vi "ISO8601 DateString to Timestamp.vi"(9 "Strict ISO? (T)":bool=TRUE, 11 "ISO8601 Date String":string) -> (1 "valid?":bool, 2 "ISO Format":T1, 3 "Timestamp":timestamp)   [LabVIEW 2018]
uses:
  ISO8601 Date Formats.ctl
  <vilib>/Utility/miscctls.llb/LVDateTimeRec.ctl
  Timestamp to ISO8601 Day.vi
  isLeapYear (integer).vi
  <vilib>/regexp/Match Regular Expression.xnode
  DateTime.ISO8601.lvclass
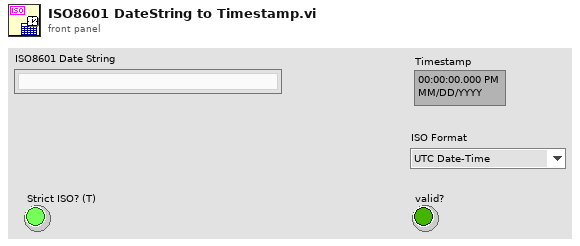
[diagram p1: front panel]
types:
  T1 = typedef "ISO8601 Date Formats.ctl" = enum16{"UTC Date-Time", "Date", "Calendar Month", "Week", "Week-Day", "Month-Day", "Ordinal Date"}
  T2 = typedef "LVDateTimeRec.ctl" = cluster{"fractional second":dbl, "second":i32, "minute":i32, "hour":i32, "day of month":i32, "month":i32, "year":i32, "day of week":i32, "day of year":i32, "DST":i32}
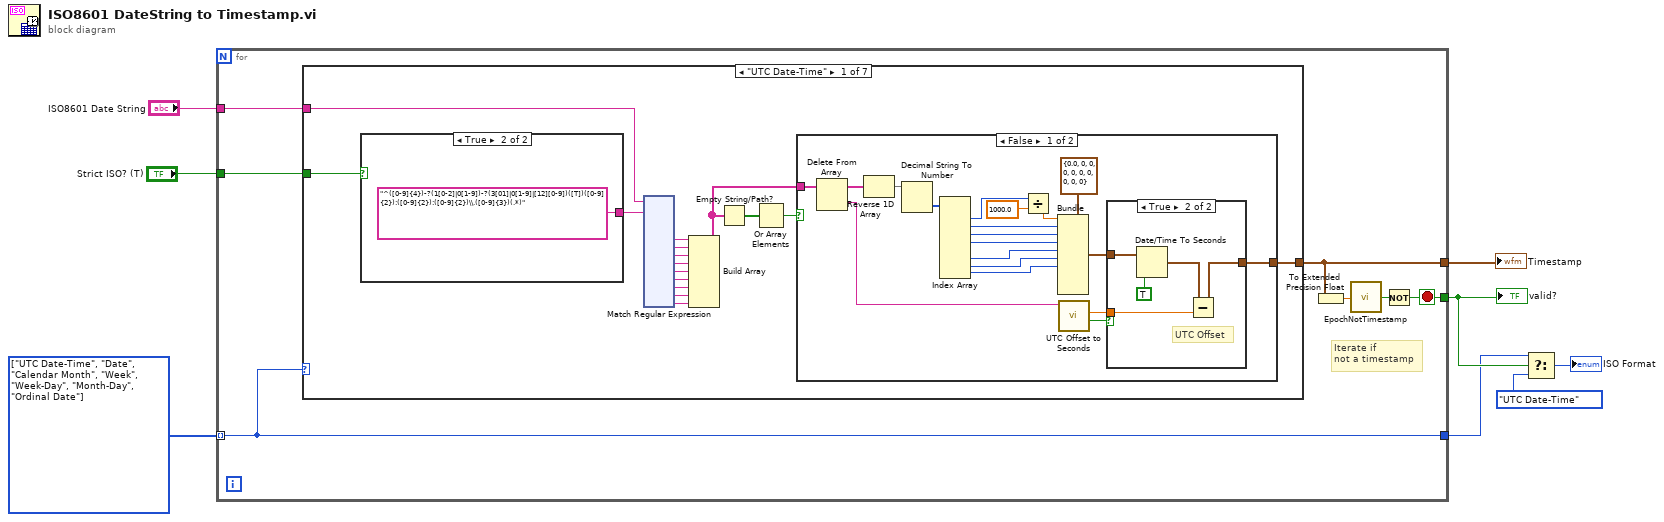
[diagram p0: block diagram]
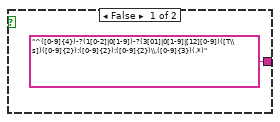
[diagram p4: hidden frame]
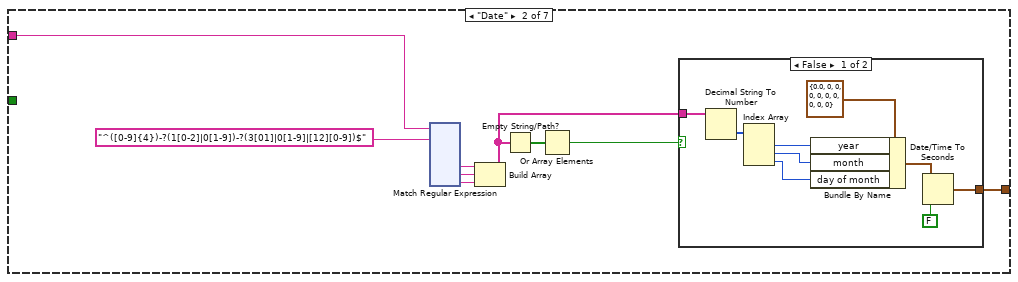
[diagram p5: hidden frame]
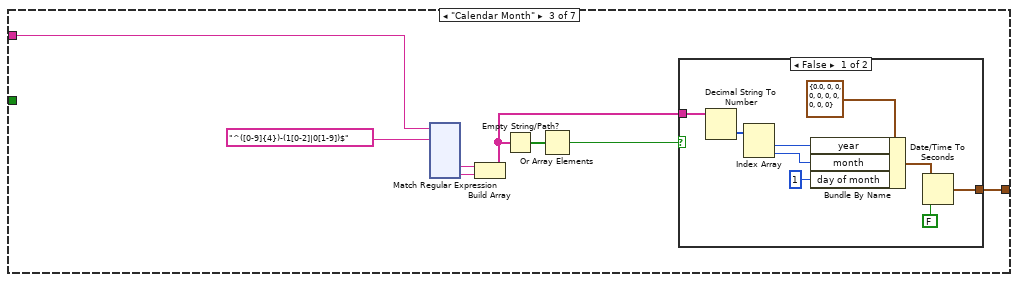
[diagram p7: hidden frame]
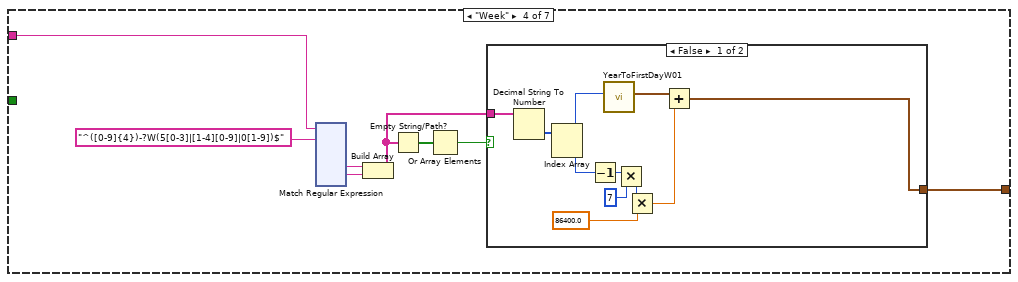
[diagram p9: hidden frame]
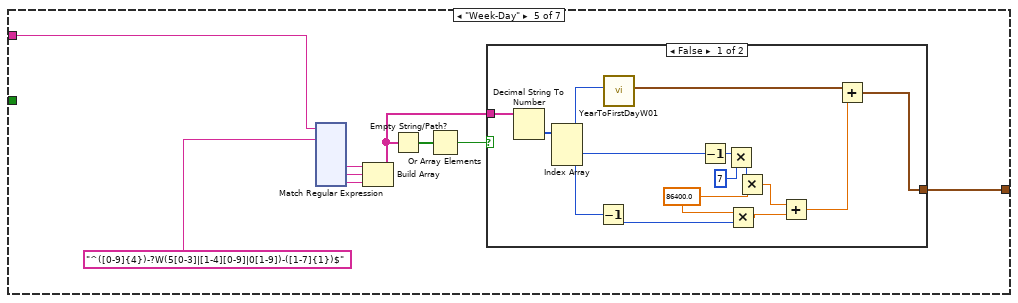
[diagram p11: hidden frame]
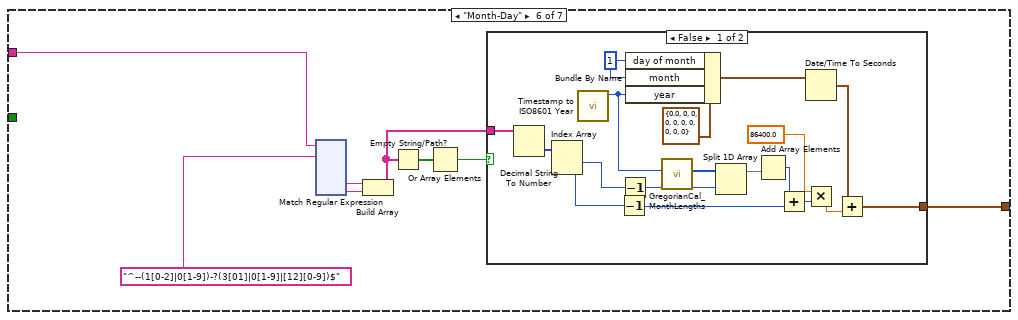
[diagram p13: hidden frame]
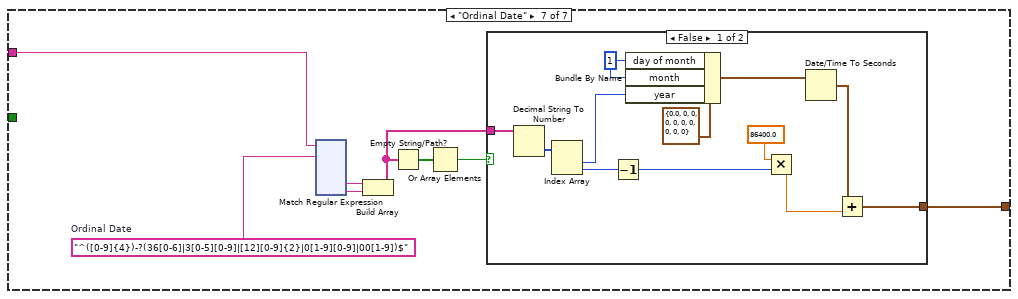
[diagram p15: hidden frame]
diagram:
  w6 = T1[] [enum."UTC Date-Time", enum."Date", enum."Calendar Month", enum."Week", enum."Week-Day", enum."Month-Day", enum."Ordinal Date"] items=["UTC Date-Time", "Date", "Calendar Month", "Week", "Week-Day", "Month-Day", "Ordinal Date"]
  n1 = for {
    tunnel: "ISO8601 Date String" -> [w15]
    tunnel: [w14] -> w7
    tunnel: [w11] -> w5
    tunnel: [w10] -> w4
    tunnel: w6 -> [w10] mode=indexing
    tunnel: "Strict ISO? (T)" -> [w9]
    stop <- w11 stop-if-true
    # "Iterate if\nnot a timestamp"
    n2 = case shown="\"UTC Date-Time\"" w10 {
      tunnel: w15 -> [w18 w184 w320 w454 w592 w733 w876]
      tunnel: w9 -> [w31 _ _ _ _ _ _]
      tunnel: [w30 w190 w325 w459 w597 w738 w881] -> w14
      frame "UTC Date-Time" {
        n3 = case shown="True" w31 {
          tunnel: ["^([0-9]{4})-?(1[0-2]|0[1-9])-?(3[01]|0[1-9]|[12][0-9])([T\\s])([0-9]{2}):([0-9]{2}):([0-9]{2})\\.([0-9]{3})(.*)" ("regular expression") "^([0-9]{4})-?(1[0-2]|0[1-9])-?(3[01]|0[1-9]|[12][0-9])([T])([0-9]{2}):([0-9]{2}):([0-9]{2})\\.([0-9]{3})(.*)" ("regular expression")] -> w17
          frame False {
          }
          frame True {
          }
        }
        n4 = xnode "Match Regular Expression"("input string"=w18, "regular expression"=w17) -> ("submatch 1"=w29:string, "submatch 2"=w28:string, "submatch 3"=w27:string, "submatch 4"=w26:string, "submatch 5"=w25:string, "submatch 6"=w24:string, "submatch 7"=w23:string, "submatch 8"=w22:string, "submatch 9"=w21:string)  [unwired: 4 in, 5 out]
        n5 = Build Array(w29, w28, w27, w26, w25, w24, w23, w22, w21) -> (w16:string[])
        n6 = Empty String/Path?(string/path=w16) -> (empty?=w20:bool[])
        n7 = Or Array Elements(Boolean array=w20) -> (logical OR=w19:bool)
        n8 = case shown="False" w19 {
          tunnel: [w174 _] -> w30
          tunnel: w16 -> [w170 _]
          frame False {
            n9 = Delete From Array(array=w170) -> (deleted portion=w168:string, array with subset deleted=w169:string[])  [unwired: 2 in]
            n10 = Reverse 1D Array(array=w169) -> (reversed array=w171:string[])
            n11 = Decimal String To Number(string=w171) -> (number=w172:i32[])  [unwired: 2 in, 1 out]
            n12 = Index Array(array=w172) -> (element #1=w164:i32, element #2=w161:i32, element #3=w160:i32, element #4=w159:i32, element #6=w158:i32, element #7=w157:i32, element #8=w156:i32)  [unwired: 8 in, 1 out]
            n13 = Divide(x=w164, y=1000.0) -> (x/y=w162:dbl)
            n14 = Bundle(cluster=T2 {"fractional second"=0.0, "second"=0, "minute"=0, "hour"=0, "day of month"=0, "month"=0, "year"=0, "day of week"=0, "day of year"=0, "DST"=0} ("date time rec"), "fractional second"=w162, "second"=w161, "minute"=w160, "hour"=w159, "day of month"=w158, "month"=w157, "year"=w156) -> (w165:T2)  [unwired: 3 in]
            n15 = call "UTC Offset to Seconds.vi"("UTC Offset String"=w168) -> ("Valid?"=w166:bool, "Offset (s)"=w167:ext)  [unwired: 8 in, 1 out]
            n16 = case shown="True" w166 {
              tunnel: w165 -> [_ w178]
              tunnel: w167 -> [_ w177]
              tunnel: [_ w176] -> w174
              frame False {
              }
              frame True {
                # "UTC Offset"
                n17 = Date/Time To Seconds(1:TRUE ("is UTC (F)"), 2:w178) -> (0:w175:timestamp)
                n18 = Subtract(x=w175, y=w177) -> (x-y=w176:timestamp)
              }
            }
          }
          frame True {
          }
        }
      }
      frame "Date" {
        n19 = xnode "Match Regular Expression"("input string"=w184, "regular expression"="^([0-9]{4})-?(1[0-2]|0[1-9])-?(3[01]|0[1-9]|[12][0-9])$") -> ("submatch 1"=w189:string, "submatch 2"=w188:string, "submatch 3"=w187:string)  [unwired: 4 in, 5 out]
        n20 = Build Array(w189, w188, w187) -> (w182:string[])
        n21 = Empty String/Path?(string/path=w182) -> (empty?=w186:bool[])
        n22 = Or Array Elements(Boolean array=w186) -> (logical OR=w185:bool)
        n23 = case shown="False" w185 {
          tunnel: [w317 _] -> w190
          tunnel: w182 -> [w313 _]
          frame False {
            n24 = Decimal String To Number(string=w313) -> (number=w315:i32[])  [unwired: 2 in, 1 out]
            n25 = Index Array(array=w315) -> (element #1=w312:i32, element #2=w311:i32, element #3=w310:i32)  [unwired: 3 in]
            n26 = Bundle By Name(cluster=T2 {"fractional second"=0.0, "second"=0, "minute"=0, "hour"=0, "day of month"=0, "month"=0, "year"=0, "day of week"=0, "day of year"=0, "DST"=0} ("date time rec"), "year"=w312, "month"=w311, "day of month"=w310) -> (w309:T2)
            n27 = Date/Time To Seconds(1:FALSE ("is UTC (F)"), 2:w309) -> (0:w317:timestamp)
          }
          frame True {
          }
        }
      }
      frame "Calendar Month" {
        n28 = xnode "Match Regular Expression"("input string"=w320, "regular expression"="^([0-9]{4})-(1[0-2]|0[1-9])$") -> ("submatch 1"=w324:string, "submatch 2"=w323:string)  [unwired: 4 in, 5 out]
        n29 = Build Array(w324, w323) -> (w318:string[])
        n30 = Empty String/Path?(string/path=w318) -> (empty?=w322:bool[])
        n31 = Or Array Elements(Boolean array=w322) -> (logical OR=w321:bool)
        n32 = case shown="False" w321 {
          tunnel: [w451 _] -> w325
          tunnel: w318 -> [w447 _]
          frame False {
            n33 = Decimal String To Number(string=w447) -> (number=w449:i32[])  [unwired: 2 in, 1 out]
            n34 = Index Array(array=w449) -> (element #1=w446:i32, element #2=w445:i32)  [unwired: 2 in]
            n35 = Bundle By Name(cluster=T2 {"fractional second"=0.0, "second"=0, "minute"=0, "hour"=0, "day of month"=0, "month"=0, "year"=0, "day of week"=0, "day of year"=0, "DST"=0} ("date time rec"), "year"=w446, "month"=w445, "day of month"=1) -> (w444:T2)
            n36 = Date/Time To Seconds(1:FALSE ("is UTC (F)"), 2:w444) -> (0:w451:timestamp)
          }
          frame True {
          }
        }
      }
      frame "Week" {
        n37 = xnode "Match Regular Expression"("input string"=w454, "regular expression"="^([0-9]{4})-?W(5[0-3]|[1-4][0-9]|0[1-9])$") -> ("submatch 1"=w458:string, "submatch 2"=w457:string)  [unwired: 4 in, 6 out]
        n38 = Build Array(w458, w457) -> (w452:string[])
        n39 = Empty String/Path?(string/path=w452) -> (empty?=w456:bool[])
        n40 = Or Array Elements(Boolean array=w456) -> (logical OR=w455:bool)
        n41 = case shown="False" w455 {
          tunnel: [w578 _] -> w459
          tunnel: w452 -> [w587 _]
          frame False {
            n42 = Decimal String To Number(string=w587) -> (number=w588:i32[])  [unwired: 2 in, 1 out]
            n43 = Index Array(array=w588) -> (element #1=w586:i32, element #2=w585:i32)  [unwired: 2 in]
            n44 = Decrement(x=w585) -> (x-1=w584:i32)
            n45 = call "YearToFirstDayW01.vi"("year"=w586) -> ("First Day of W01"=w580:timestamp)  [unwired: 10 in]
            n46 = Multiply(x=w584, y=7) -> (x*y=w583:i32)
            n47 = Multiply(x=w583, y=86400.0) -> (x*y=w579:dbl)
            n48 = Add(x=w580, y=w579) -> (x+y=w578:timestamp)
          }
          frame True {
          }
        }
      }
      frame "Week-Day" {
        n49 = xnode "Match Regular Expression"("input string"=w592, "regular expression"="^([0-9]{4})-?W(5[0-3]|[1-4][0-9]|0[1-9])-([1-7]{1})$") -> ("submatch 1"=w596:string, "submatch 2"=w595:string, "submatch 3"=w590:string)  [unwired: 4 in, 5 out]
        n50 = Build Array(w596, w595, w590) -> (w591:string[])
        n51 = Empty String/Path?(string/path=w591) -> (empty?=w594:bool[])
        n52 = Or Array Elements(Boolean array=w594) -> (logical OR=w593:bool)
        n53 = case shown="False" w593 {
          tunnel: [w722 _] -> w597
          tunnel: w591 -> [w729 _]
          frame False {
            w718 = 86400.0
            n54 = Decimal String To Number(string=w729) -> (number=w730:i32[])  [unwired: 2 in, 1 out]
            n55 = Index Array(array=w730) -> (element #1=w728:i32, element #2=w727:i32, element #3=w719:i32)  [unwired: 3 in]
            n56 = Decrement(x=w719) -> (x-1=w717:i32)
            n57 = call "YearToFirstDayW01.vi"("year"=w728) -> ("First Day of W01"=w723:timestamp)  [unwired: 10 in]
            n58 = Decrement(x=w727) -> (x-1=w726:i32)
            n59 = Multiply(x=w726, y=7) -> (x*y=w725:i32)
            n60 = Multiply(x=w718, y=w717) -> (x*y=w716:dbl)
            n61 = Multiply(x=w725, y=w718) -> (x*y=w721:dbl)
            n62 = Add(x=w721, y=w716) -> (x+y=w720:dbl)
            n63 = Add(x=w723, y=w720) -> (x+y=w722:timestamp)
          }
          frame True {
          }
        }
      }
      frame "Month-Day" {
        n64 = xnode "Match Regular Expression"("input string"=w733, "regular expression"="^--(1[0-2]|0[1-9])-?(3[01]|0[1-9]|[12][0-9])$") -> ("submatch 1"=w737:string, "submatch 2"=w736:string)  [unwired: 4 in, 5 out]
        n65 = Build Array(w737, w736) -> (w732:string[])
        n66 = Empty String/Path?(string/path=w732) -> (empty?=w735:bool[])
        n67 = Or Array Elements(Boolean array=w735) -> (logical OR=w734:bool)
        n68 = case shown="False" w734 {
          tunnel: [w871 _] -> w738
          tunnel: w732 -> [w872 _]
          frame False {
            w867 = 1 ("day of month")
            n69 = Decimal String To Number(string=w872) -> (number=w873:i32[])  [unwired: 2 in, 1 out]
            n70 = Index Array(array=w873) -> (element #1=w862:i32, element #2=w870:i32)  [unwired: 2 in]
            n71 = call "Timestamp to ISO8601 Year.vi"() -> ("year"=w864:i32)  [unwired: 10 in, 1 out]
            n72 = Decrement(x=w870) -> (x-1=w858:i32)
            n73 = Decrement(x=w862) -> (x-1=w861:i32)
            n74 = Bundle By Name(cluster=T2 {"fractional second"=0.0, "second"=0, "minute"=0, "hour"=0, "day of month"=0, "month"=0, "year"=0, "day of week"=0, "day of year"=0, "DST"=0} ("date time rec"), "day of month"=w867, "month"=w867, "year"=w864) -> (w868:T2)
            n75 = call "GregorianCal_MonthLengths.vi"("Year (0: this year)"=w864) -> ("Month Lengths"=w863:i32[])  [unwired: 10 in]
            n76 = Split 1D Array(array=w863, index=w861) -> (first subarray=w860:i32[])  [unwired: 1 out]
            n77 = Add Array Elements(numeric array=w860) -> (sum=w859:i32)
            n78 = Add(x=w859, y=w858) -> (x+y=w857:i32)
            n79 = Date/Time To Seconds(2:w868) -> (0:w865:timestamp)  [unwired: 1 in]
            n80 = Multiply(x=86400.0, y=w857) -> (x*y=w856:dbl)
            n81 = Add(x=w865, y=w856) -> (x+y=w871:timestamp)
          }
          frame True {
          }
        }
      }
      frame "Ordinal Date" {
        w874 = "^([0-9]{4})-?(36[0-6]|3[0-5][0-9]|[12][0-9]{2}|0[1-9][0-9]|00[1-9])$"  # Ordinal Date
        n82 = xnode "Match Regular Expression"("input string"=w876, "regular expression"=w874) -> ("submatch 1"=w880:string, "submatch 2"=w879:string)  [unwired: 4 in, 5 out]
        n83 = Build Array(w880, w879) -> (w875:string[])
        n84 = Empty String/Path?(string/path=w875) -> (empty?=w878:bool[])
        n85 = Or Array Elements(Boolean array=w878) -> (logical OR=w877:bool)
        n86 = case shown="False" w877 {
          tunnel: [w1008 _] -> w881
          tunnel: w875 -> [w1009 _]
          frame False {
            w1004 = 1 ("day of month")
            n87 = Decimal String To Number(string=w1009) -> (number=w1010:i32[])  [unwired: 2 in, 1 out]
            n88 = Index Array(array=w1010) -> (element #1=w1000:i32, element #2=w1007:i32)  [unwired: 2 in]
            n89 = Decrement(x=w1007) -> (x-1=w999:i32)
            n90 = Bundle By Name(cluster=T2 {"fractional second"=0.0, "second"=0, "minute"=0, "hour"=0, "day of month"=0, "month"=0, "year"=0, "day of week"=0, "day of year"=0, "DST"=0} ("date time rec"), "day of month"=w1004, "month"=w1004, "year"=w1000) -> (w1005:T2)
            n91 = Multiply(x=86400.0, y=w999) -> (x*y=w1001:dbl)
            n92 = Date/Time To Seconds(2:w1005) -> (0:w1002:timestamp)  [unwired: 1 in]
            n93 = Add(x=w1002, y=w1001) -> (x+y=w1008:timestamp)
          }
          frame True {
          }
        }
      }
    }
    n94 = To Extended Precision Float(1:w14) -> (0:w13:ext)
    n95 = call "EpochNotTimestamp.vi"("Epoch Time"=w13) -> ("Not a Timestamp?"=w12:bool)  [unwired: 8 in]
    n96 = Not(x=w12) -> (.not. x?=w11:bool)
  }
  "Timestamp" <- w7
  "valid?" <- w5
  n97 = Select(t=w4, s=w5, f=ISO8601_Date_Formats."UTC Date-Time" ("ISO Format")) -> (s? t:f=→"ISO Format":T1)
